vi "Firma.vi"() -> ()   [LabVIEW 2016]
uses:
  <vilib>/Utility/miscctls.llb/LVMouseTypeDef.ctl
panel:
  out "XY Graph":cluster{i32[], i32[]}(graph)
  out "Waveform Graph 2":i32[](graph)
  out "Waveform Graph":i32[](graph)
  out "Mouse":T1
  in  "Stop Button":bool
  out "2D Picture":picture
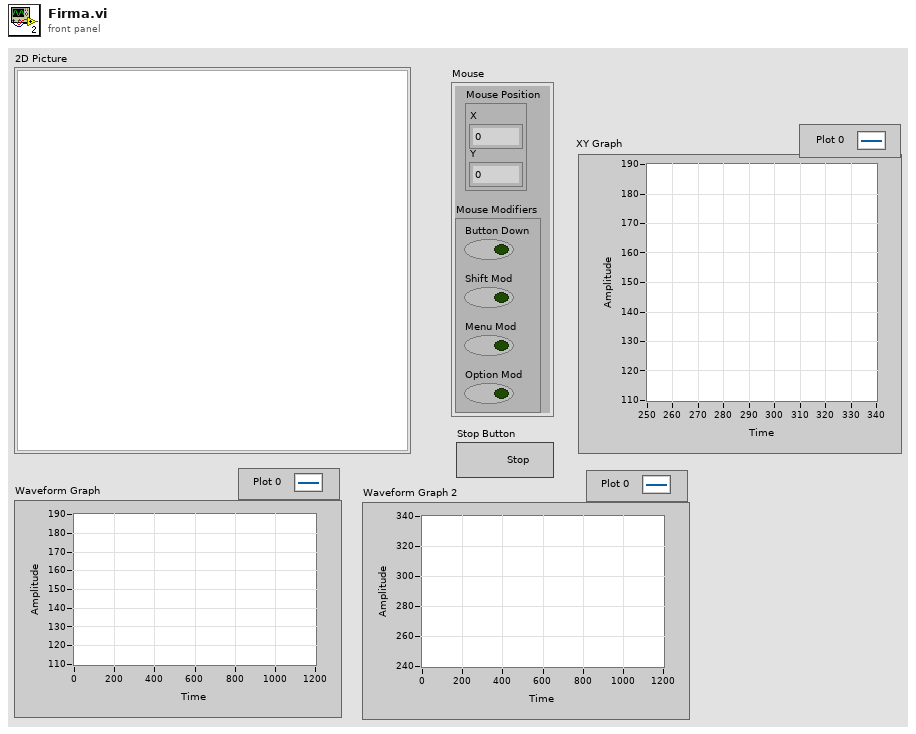
[diagram p1: front panel]
types:
  T1 = typedef "LVMouseTypeDef.ctl" = cluster{"Mouse Position":cluster{"X":i32, "Y":i32}, "Mouse Modifiers":cluster{"Button Down":bool, "Shift Mod":bool, "Menu Mod":bool, "Option Mod":bool}}
  T2 = cluster{"Width":u16, "Style":enum32{"Solid", "Dash", "Dot", "DashDot", "DashDotDot"}}
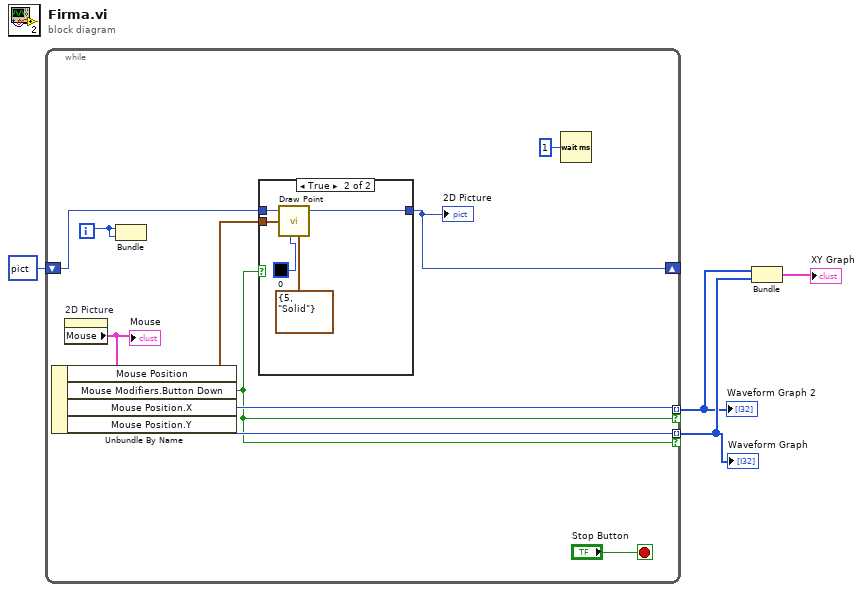
[diagram p0: block diagram]
diagram:
  n1 = while {
    shift-right: [w12] -> _
    shift-left: picture data[5B] ("new picture") -> [w11]
    tunnel: [w7] -> w1 mode=indexing if=w5
    tunnel: [w6] -> w2 mode=indexing if=w5
    i -> [w14]
    stop <- "Stop Button" stop-if-true
    n2 = property on="2D Picture" class="Pict"() -> ("Mouse"=w9:T1)  [unwired: 2 in, 2 out]
    "Mouse" <- w9
    n3 = Unbundle By Name(w9) -> ("Mouse Position"=w8:cluster{"X":i32, "Y":i32}, "Mouse Modifiers.Button Down"=w5:bool, "Mouse Position.X"=w7:i32, "Mouse Position.Y"=w6:i32)
    n4 = Bundle(w14, w14) -> ()  [unwired: 1 in, 1 out]
    n5 = case shown="True" w5 {
      tunnel: [w15 w19] -> w12
      tunnel: w11 -> [w15 w18]
      tunnel: w8 -> [_ w17]
      frame False {
      }
      frame True {
        n6 = call <vilib>:"Draw Point.vi"("picture"=w18, "point(x,y)"=w17, "color(black)"=u32 0, "pen"=T2 {"Width"=5, "Style"=enum."Solid"}) -> ("new picture"=w19:picture)  [unwired: 5 in]
      }
    }
    "2D Picture" <- w12
    n7 = Wait (ms)(milliseconds to wait=u32 1) -> ()  [unwired: 1 out]
  }
  "Waveform Graph" <- w2
  "Waveform Graph 2" <- w1
  n8 = Bundle(w1, w2) -> (→"XY Graph":cluster{i32[], i32[]})  [unwired: 1 in]
